vi "Check_EnFlo_Arm.vi"() -> ()   [LabVIEW 2012]
uses:
  Gen Trav/Trav_mode.ctl
  Gen Trav/Route mapping/Route_mapping_global.vi
  Globals/Trav_pos_global.vi
  ADAM Serial/Instrument drivers/Traverses/~subVIs/DriveConfigGlobal.vi
panel:
  out "Position Output XYZ":dbl[](array[numeric]) format="%.2f"
  in  "Mode":T1(ring)
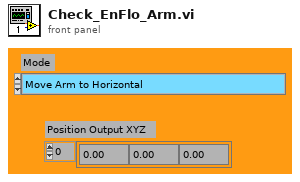
[diagram p1: front panel]
types:
  T1 = enum16{"Move Arm to Horizontal", "Teach Traverse That Arm is Level"}
  T2 = typedef "Tunnel_Coordinates.ctl" = enum16{"Work in Tunnel Coordinates", "Work in Model Coordinates"}
  T3 = typedef "Box_size.ctl" = cluster{"Max":dbl, "Min":dbl}[]
  T4 = typedef "Exclude_cluster.ctl" = cluster{"Sizes":T3, "Name":string, "Exclude Type":T5}
  T5 = typedef "Exclusion_type.ctl" = enum16{"Exclude completely", "Allow only vertical moves"}
  T6 = typedef "Trav_mode.ctl" = enum16{"Move traverse", "Read traverse position", "Teach Position"}
  T7 = enum16{"Load setup from excel file", "Save setup to excel file"}
  T8 = typedef "AxisConfigCluster.ctl" = cluster{"Channel Properties":T9, "Static Drive Configuration":T10}
  T9 = typedef "DriveProperties.ctl" = cluster{"Channel Name":string, "Vel. Default":dbl, "Acc. Default":dbl, "Vel. Max":dbl, "Vel. Min":dbl, "Acc. Max":dbl, "Acc. Min":dbl, "Pulses/unit":dbl, "Address":u8, "Pulse Offset":i32, "Pos Tolerance":dbl, "Pulses/rev":dbl, "Backlash/Eng units":dbl, "Current Pos":dbl, "Ch Status":enum16{"Active", "Offline", "Simulate"}, "Port Name":string, "Axis Transform mode":string, "Metadata Ch Name":string, "Type":string}
  T10 = typedef "DriveStaticConfig.ctl" = cluster{"Correction Gain % (CG)":u16, "Dead Band (DB)":i32, "Dead Band Window (DW)":i32, "Encoder Resolution (ER)":i32, "Step Mode  (FSB)":u16, "Position Maintenance (FSC)":u16, "Stop on Stall (FSD)":u16, "Activate OP1 on stall (FSE)":u16, "Stop on Trigger 3 (FSF)":u16, "OP2 in Deadband (FSG)":u16, "Stall Detect (FSH)":u16, "Limit Disable (LD)":u16, "Motor Resolution (MR)":enum16{"200", "400", "1000", "2000", "4000", "5000", "10000", "12800", "18000", "20000", "21600", "25000", "25400", "25600", "36000", "50000", "278528", "425984", "507904", "614400", "655360", "819200", "1024000"}, "Limit Switch Sense (OSA)":u16, "Home Position (OSB)":u16, "Home Switch Sense (OSC)":u16, "Encoder Z for Home (OSD)":u16, "Reference edge of Home (OSH)":u16, "RS232 Echo Control (SSA)":u16, "Buffer at Limit (SSG)":u16, "Buffer at Stop (SSH)":u16, "Indexer Mode  (FSA)":u16, "Type":string, "ConfigString":string, "De Power Motor":enum16{"TRUE", "FALSE"}}
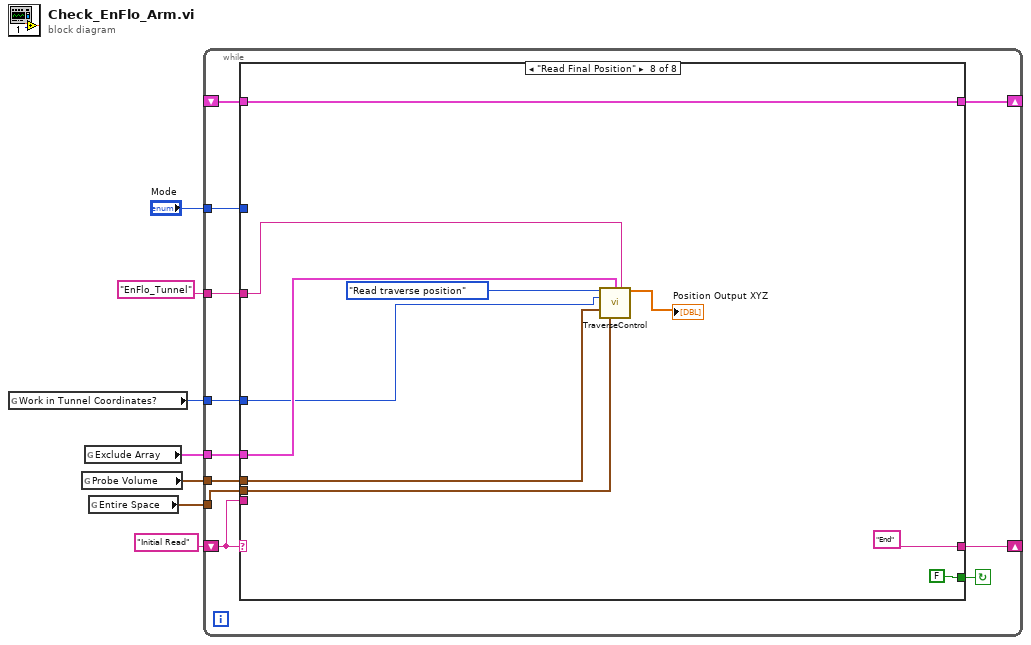
[diagram p0: block diagram]
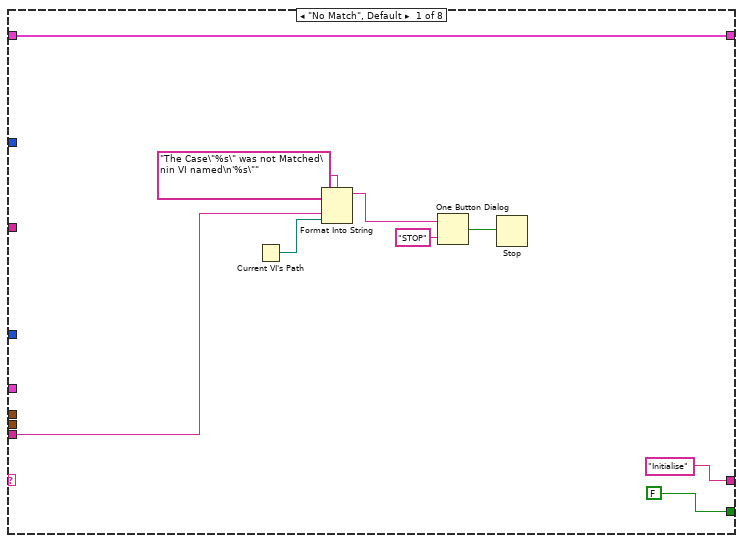
[diagram p2: hidden frame]
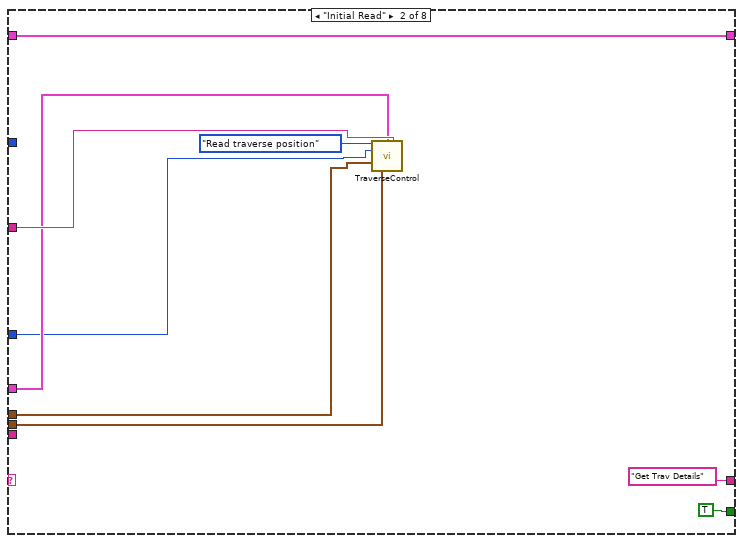
[diagram p3: hidden frame]
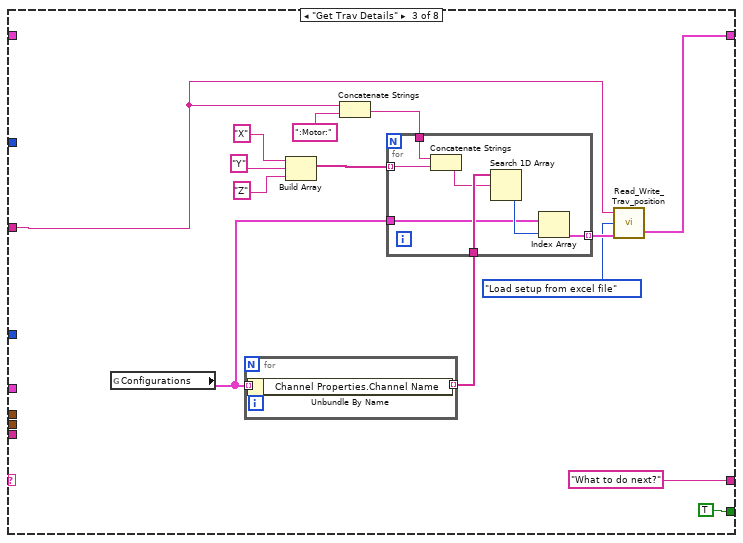
[diagram p4: hidden frame]
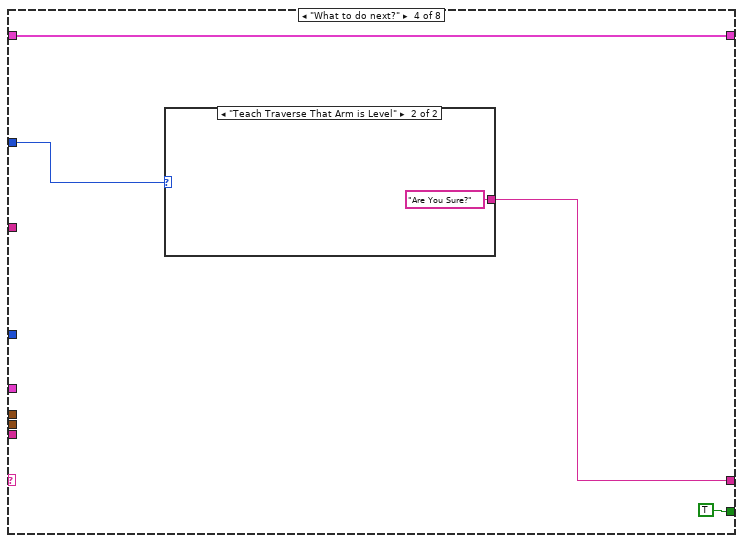
[diagram p5: hidden frame]
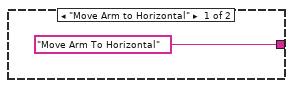
[diagram p6: hidden frame]
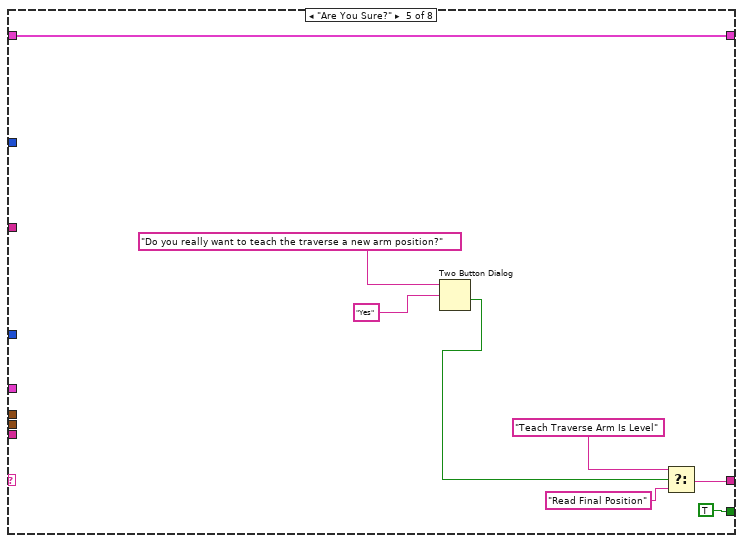
[diagram p7: hidden frame]
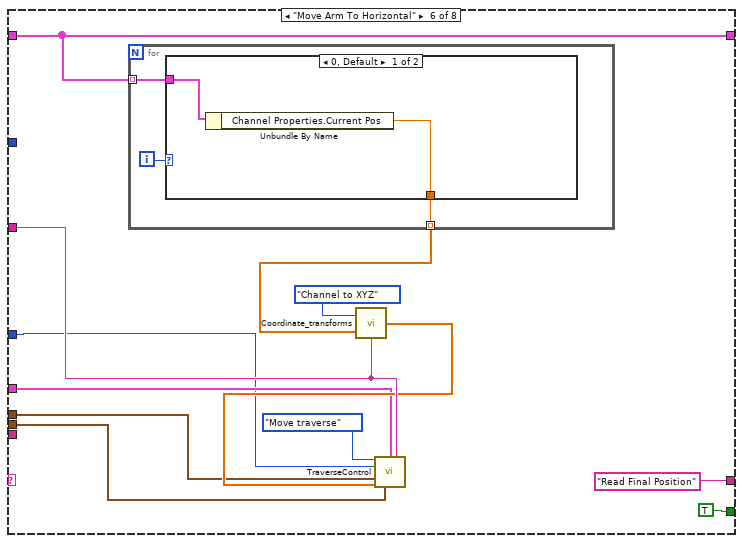
[diagram p8: hidden frame]
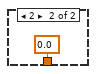
[diagram p9: hidden frame]
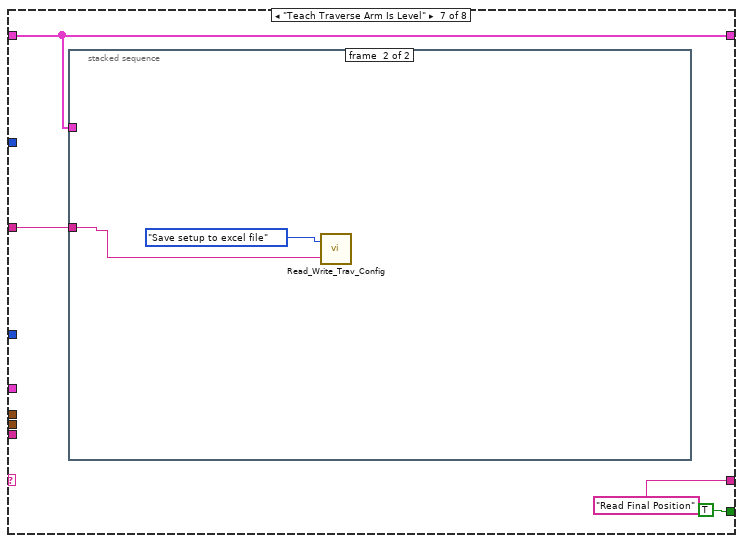
[diagram p10: hidden frame]
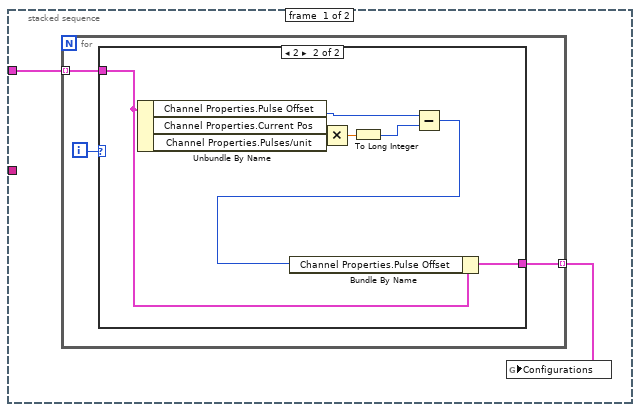
[diagram p11: hidden frame]
diagram:
  n1 = global read "Trav_pos_global.vi" "Work in Tunnel Coordinates?"() -> (w1:T2)
  n2 = global read "Route_mapping_global.vi" "Probe Volume"() -> (w3:T3)
  n3 = global read "Route_mapping_global.vi" "Exclude Array"() -> (w4:T4[])
  n4 = global read "Route_mapping_global.vi" "Entire Space"() -> (w2:T3)
  n5 = while {
    tunnel: "Mode" -> [w12]
    shift-left: _ -> [w13]
    shift-right: [w14] -> _
    tunnel: "EnFlo_Tunnel" ("Traverse Name") -> [w15]
    shift-left: "Initial Read" -> [w16]
    shift-right: [w17] -> _
    tunnel: w4 -> [w11]
    tunnel: w3 -> [w10]
    tunnel: w2 -> [w9]
    tunnel: w1 -> [w8]
    stop <- w18 continue-if-true
    n6 = case shown="\"Read Final Position\"" w16 {
      tunnel: [FALSE TRUE TRUE TRUE TRUE TRUE TRUE FALSE] -> w18
      tunnel: ["Initialise" "Get Trav Details" "What to do next?" w61 w67 "Read Final Position" "Read Final Position" "End"] -> w17
      tunnel: w16 -> [w22 _ _ _ _ _ _ _]
      tunnel: w15 -> [_ w32 w38 _ _ w80 w92 w118]
      tunnel: [w19 w33 w37 w60 w72 w83 w93 w117] -> w14
      tunnel: w13 -> [w19 w33 _ w60 w72 w83 w93 w117]
      tunnel: w12 -> [_ _ _ w62 _ _ _ _]
      tunnel: w11 -> [_ w31 _ _ _ w77 _ w115]
      tunnel: w10 -> [_ w29 _ _ _ w76 _ w113]
      tunnel: w9 -> [_ w30 _ _ _ w75 _ w114]
      tunnel: w8 -> [_ w28 _ _ _ w74 _ w112]
      frame "No Match", Default {
        n7 = Current VI's Path() -> (path=w21:path)
        n8 = Format Into String(format string="The Case\"%s\" was not Matched\nin VI named\n'%s\"" ("Format String"), w22, w21) -> (resulting string=w25:string)  [unwired: 2 in, 1 out]
        n9 = One Button Dialog(message=w25, button name ("OK")="STOP") -> (true=w23:bool)
        n10 = Stop(stop? (T)=w23) -> ()
      }
      frame "Initial Read" {
        n11 = call "TraverseControl.vi"("Mode"=Trav_mode."Read traverse position", "Exclude Array"=w31, "Traverse Name"=w32, "Work in Tunnel Coordinates?"=w28, "Probe Volume"=w29, "Entire Space"=w30) -> ()  [unwired: 8 in, 2 out]
      }
      frame "Get Trav Details" {
        n12 = global read "DriveConfigGlobal.vi" "Configurations"() -> (w41:T8[])
        n13 = for {
          tunnel: w41 -> [w52] mode=indexing
          tunnel: [w51] -> w42 mode=indexing
          n14 = Unbundle By Name(w52) -> ("Channel Properties.Channel Name"=w51:string)
        }
        n15 = Build Array("X", "Y", "Z") -> (w47:string[])
        n16 = Concatenate Strings(w38, ":Motor:") -> (w46:string)
        n17 = for {
          tunnel: w47 -> [w59] mode=indexing
          tunnel: w46 -> [w58]
          tunnel: w42 -> [w57]
          tunnel: w41 -> [w54]
          tunnel: [w53] -> w40 mode=indexing
          n18 = Concatenate Strings(w58, w59) -> (w56:string)
          n19 = Search 1D Array(1D array=w57, element=w56) -> (index of element=w55:i32)  [unwired: 1 in]
          n20 = Index Array(array=w54, index=w55) -> (element=w53:T8)
        }
        n21 = call "Read_Write_Trav_position.vi"("Matched Configurations In"=w40, "Mode"=T7."Load setup from excel file", "Traverse Name"=w38) -> ("Matched Configurations Out"=w37:T8[])  [unwired: 1 in]
      }
      frame "What to do next?" {
        n22 = case shown="\"Teach Traverse That Arm is Level\"" w62 {
          tunnel: ["Move Arm To Horizontal" "Are You Sure?"] -> w61
          frame "Move Arm to Horizontal" {
          }
          frame "Teach Traverse That Arm is Level" {
          }
        }
      }
      frame "Are You Sure?" {
        n23 = Two Button Dialog(message="Do you really want to teach the traverse a new arm position?", 2:"Yes" ("T button name (\"OK\")")) -> (T button?=w69:bool)  [unwired: 1 in]
        n24 = Select(t="Teach Traverse Arm Is Level", s=w69, f="Read Final Position") -> (s? t:f=w67:string)
      }
      frame "Move Arm To Horizontal" {
        n25 = for {
          tunnel: w83 -> [w87] mode=indexing
          tunnel: [w86] -> w81 mode=indexing
          i -> [w88]
          n26 = case shown="0, Default" w88 {
            tunnel: w87 -> [w90 _]
            tunnel: [w89 0.0 ("Current Pos")] -> w86
            frame 0, Default {
              n27 = Unbundle By Name(w90) -> ("Channel Properties.Current Pos"=w89:dbl)
            }
            frame 2 {
            }
          }
        }
        n28 = call "Coordinate_transforms.vi"("Traverse Name"=w80, "Input"=w81, "Mode"=enum16{"XYZ to Channel", "Channel to XYZ"}."Channel to XYZ") -> ("Output"=w79:dbl[])
        n29 = call "TraverseControl.vi"("Mode"=Trav_mode."Move traverse", "Exclude Array"=w77, "Traverse Name"=w80, "Work in Tunnel Coordinates?"=w74, "Probe Volume"=w76, "Position input XYZ"=w79, "Entire Space"=w75) -> ()  [unwired: 7 in, 2 out]
      }
      frame "Teach Traverse Arm Is Level" {
        n30 = stacked-sequence {
          tunnel: w93 -> [w97 _]
          tunnel: w92 -> [_ w110]
          frame #0 {
            n31 = for {
              tunnel: w97 -> [w99] mode=indexing
              tunnel: [w98] -> w96 mode=indexing
              i -> [w100]
              n32 = case shown="2" w100 {
                tunnel: w99 -> [w101 w106]
                tunnel: [w101 w102] -> w98
                frame 0, Default {
                }
                frame 2 {
                  n33 = Unbundle By Name(w106) -> ("Channel Properties.Pulse Offset"=w107:i32, "Channel Properties.Current Pos"=w109:dbl, "Channel Properties.Pulses/unit"=w108:dbl)
                  n34 = Multiply(x=w109, y=w108) -> (x*y=w105:dbl)
                  n35 = To Long Integer(number=w105) -> (32bit integer=w104:i32)
                  n36 = Subtract(x=w107, y=w104) -> (x-y=w103:i32)
                  n37 = Bundle By Name(cluster=w106, "Channel Properties.Pulse Offset"=w103) -> (w102:T8)
                }
              }
            }
            n38 = global write "DriveConfigGlobal.vi" "Configurations"(w96) -> ()
          }
          frame #1 {
            n39 = call "Read_Write_Trav_Config.vi"("Traverse Name"=w110, "Mode"=T7."Save setup to excel file") -> ()  [unwired: 1 in]
          }
        }
      }
      frame "Read Final Position" {
        n40 = call "TraverseControl.vi"("Mode"=Trav_mode."Read traverse position", "Exclude Array"=w115, "Traverse Name"=w118, "Work in Tunnel Coordinates?"=w112, "Probe Volume"=w113, "Entire Space"=w114) -> ("Position Output XYZ"=→"Position Output XYZ":dbl[])  [unwired: 8 in, 1 out]
      }
    }
  }
